vi "New Connection.vi"(8 "error in (no error)":errorcluster, 9 "Timeout (5000ms)":i32=5000, 11 "Hostname / URL":string="echo.websocket.org:443") -> (0 "error out":errorcluster, 3 "dotNET TCP Socket out":refnum<class "dotNET TCP Socket.lvclass">)   [LabVIEW 2013, in "dotNET SSL Socket.lvlib" / "dotNET TCP Socket.lvclass"]
doc: "Opens a new connection to a server using .NET TCPClient."
uses:
  dotNET TCP Socket.lvclass
  <vilib>/MediaMongrels Ltd/WebSockets/WebSockets/WebSocket Client/WebSocket Client.lvclass
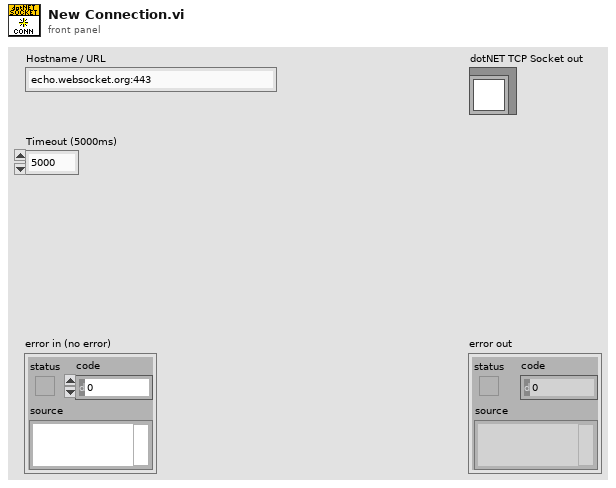
[diagram p1: front panel]
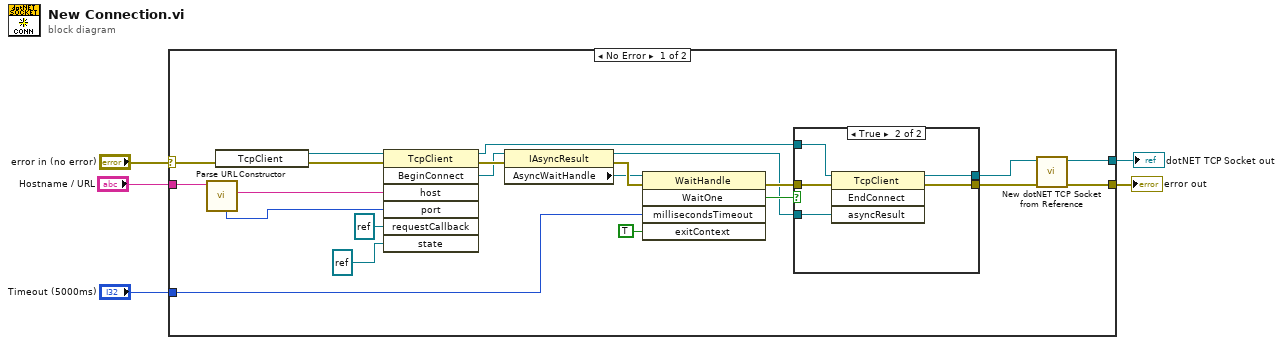
[diagram p0: block diagram]
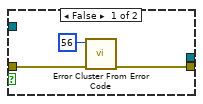
[diagram p2: hidden frame]
diagram:
  n1 = case shown="No Error" "error in (no error)" {
    selector: "error in (no error)" -> [w14 w35]
    tunnel: [w8 w35] -> w4
    tunnel: "Hostname / URL" -> [w17 _]
    tunnel: "Timeout (5000ms)" -> [w13 _]
    tunnel: [w6 _] -> w1
    frame No Error {
      n2 = call <vilib>:"Parse URL.vi"("WebSocket URL"=w17) -> ("host"=w16:string, "port"=w15:u16)  [unwired: 6 in, 3 out]
      n3 = constructor class="TcpClient"(error in=w14) -> (reference out=w20:refnum<k24>, error out=w21:errorcluster)  [unwired: 2 in, 1 out]
      n4 = invoke class="TcpClient" method="BeginConnect"(reference=w20, error in=w21, "host"=w16, "port"=w15, "requestCallback"=refnum<k24> refnum, "state"=refnum<k24> refnum) -> (reference out=w10:refnum<k24>, error out=w26:errorcluster, "BeginConnect"=w25:refnum<k24>)  [unwired: 1 in, 4 out]
      n5 = property class="IAsyncResult"(reference=w25, error in=w26) -> (reference out=w9:refnum<k24>, error out=w23:errorcluster, "AsyncWaitHandle"=w22:refnum<k24>)
      n6 = invoke class="WaitHandle" method="WaitOne"(reference=w22, error in=w23, "millisecondsTimeout"=w13, "exitContext"=TRUE) -> (error out=w11:errorcluster, "WaitOne"=w12:bool)  [unwired: 1 in, 3 out]
      n7 = case shown="True" w12 {
        tunnel: w11 -> [w28 w34]
        tunnel: [w27 w31] -> w8
        tunnel: w10 -> [_ w33]
        tunnel: w9 -> [_ w32]
        tunnel: [_ w30] -> w7
        frame False {
          n8 = call <vilib>:"Error Cluster From Error Code.vi"("error in (no error)"=w28, "error code (0)"=56) -> ("error out"=w27:errorcluster)  [unwired: 7 in]
        }
        frame True {
          n9 = invoke class="TcpClient" method="EndConnect"(reference=w33, error in=w34, "asyncResult"=w32) -> (reference out=w30:refnum<k24>, error out=w31:errorcluster)  [unwired: 1 in, 2 out]
        }
      }
      n10 = call "New dotNET TCP Socket from Reference.vi"("error in (no error)"=w8, "TcpClient"=w7) -> ("dotNET TCP Socket out"=w6:refnum<class "dotNET TCP Socket.lvclass">)  [unwired: 8 in, 1 out]
    }
    frame Error {
    }
  }
  "error out" <- w4
  "dotNET TCP Socket out" <- w1
